vi "T_CAN CONF.vi"() -> ()   [LabVIEW 2018]
uses:
  Controls/CLUSTER.ctl
  Controls/FEV_DBC CLUSTER.ctl
  Controls/DBC CLUSTER.ctl
  <resource>/objmgr/xnet.rc
panel:
  out "Signals":refnum<k21>[](array[refnum])
  in  "DBC FUNCTIONS":T1[](array[typedef])
  out "Headline":string
  in  "ADD":bool
  in  "Save Button":bool
  in  "ALL DBC FUNCTIONS":T3[](array[typedef])
  in  "DBC File Selection":refnum<k21>="CAN DATA"
  in  "MODEL SELECTION":string(combo)
  # "FUNCTIONS"
  # "FUNCTIONS"
  # "READ"
  # "WRITE"
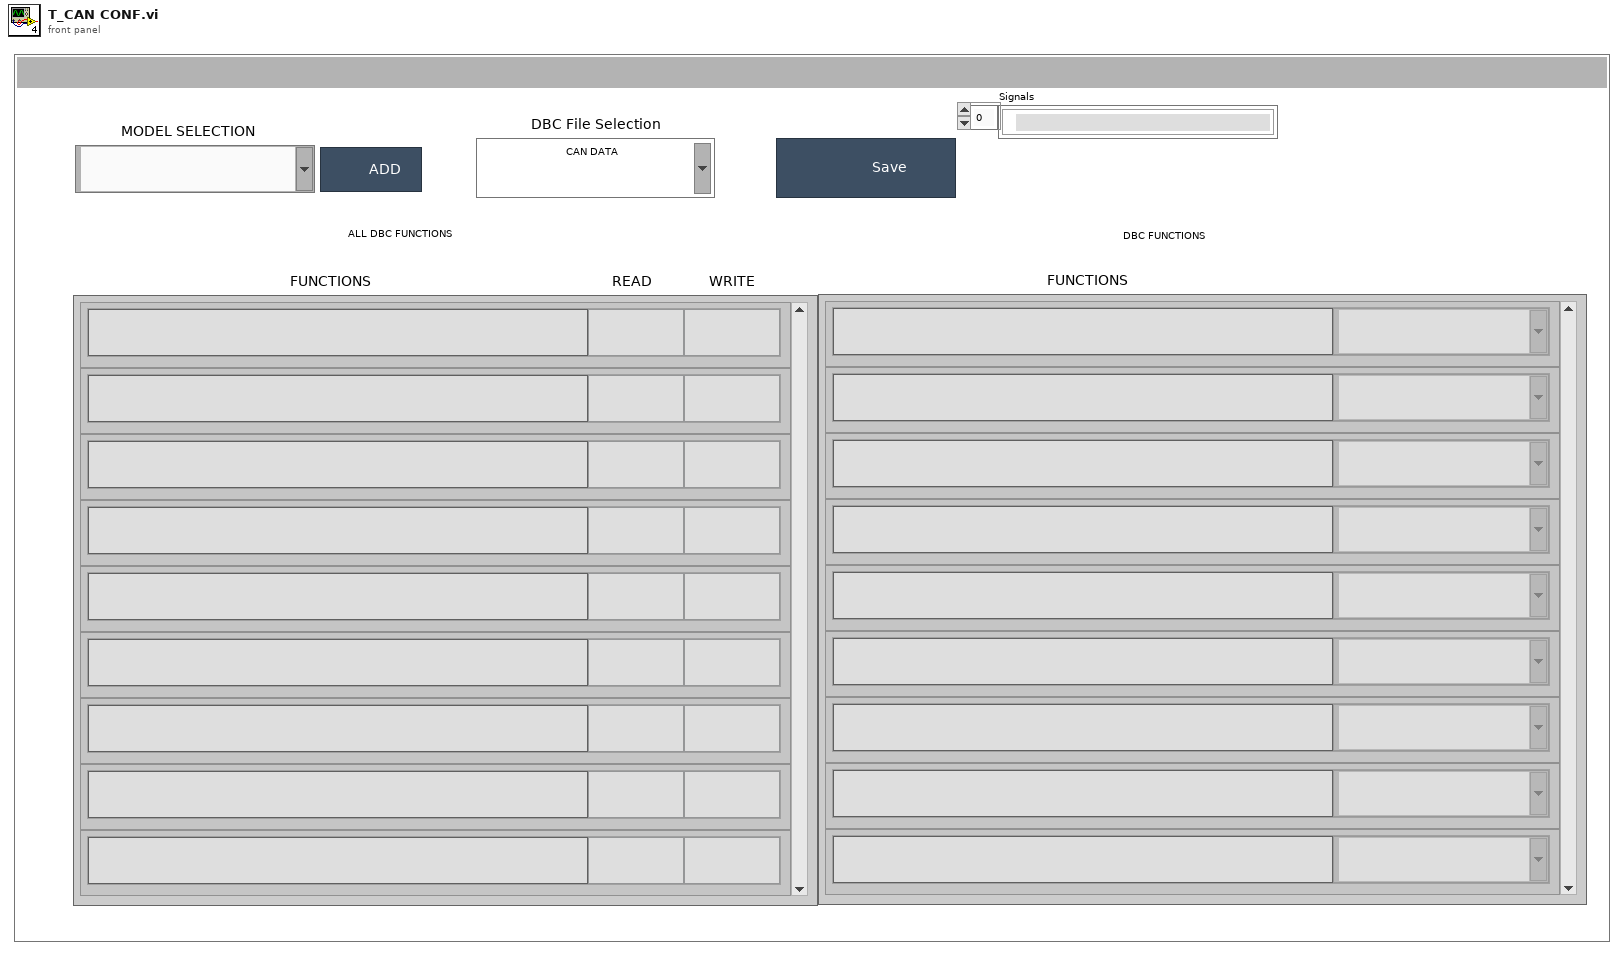
[diagram p1: front panel]
types:
  T1 = typedef "FEV_DBC CLUSTER.ctl" = cluster{"FUNCTION":T2, "DYNO FUNCTION":string}
  T2 = typedef "DBC CLUSTER.ctl" = string
  T3 = typedef "CLUSTER.ctl" = cluster{"FUNCTION":string, "READ":bool, "WRITE":bool}
  T4 = enum32{"Invalid", "Standard", "Closed", "Hidden", "Minimized", "Maximized"}
  T5 = enum32{"invalid app kind", "Development System", "Run Time System", "Student Edition", "Embedded LabVIEW", "Evaluation", "Custom"}
  T6 = cluster{"Core":cluster{"Current VI Reference":refnum<vi>, "Close Panel on Exit?":bool}, "Your Boolean data":bool, "Your string data":string, "ALL DBC FUNCTIONS":T3[], "File paths":cluster{"Base file path":path, "Model File path":path}, "DBC FUNCTIONS":T1[]}
  T7 = cluster{"Base file path":path, "Model File path":path}
  T8 = cluster{"Current VI Reference":refnum<vi>, "Close Panel on Exit?":bool}
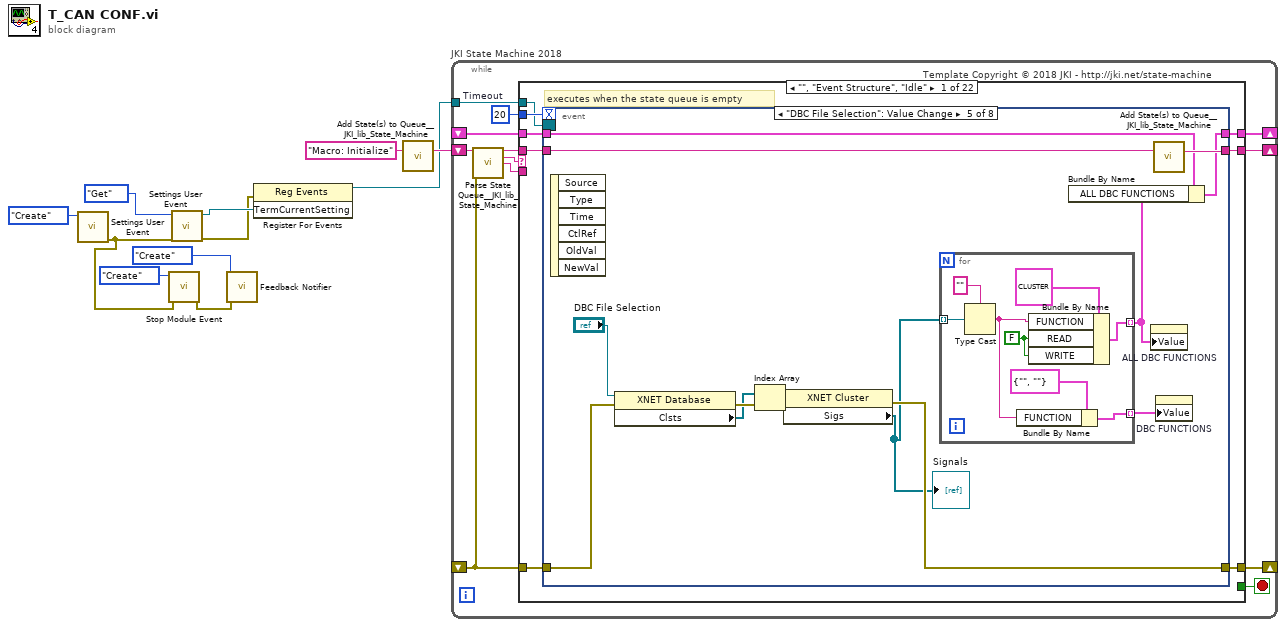
[diagram p0: block diagram]
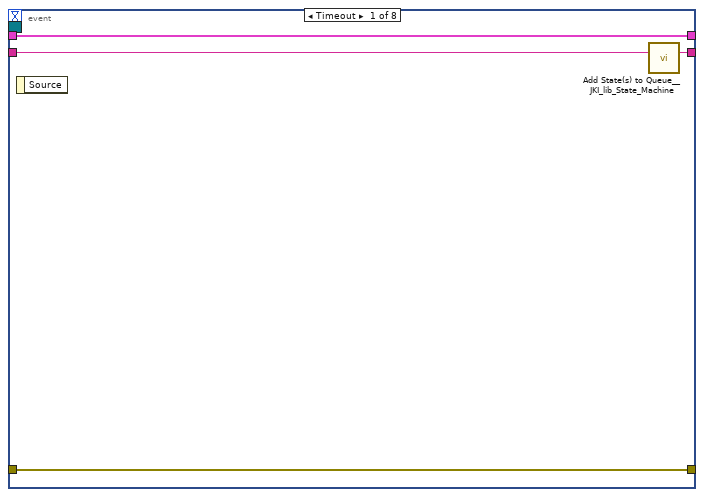
[diagram p2: hidden frame]
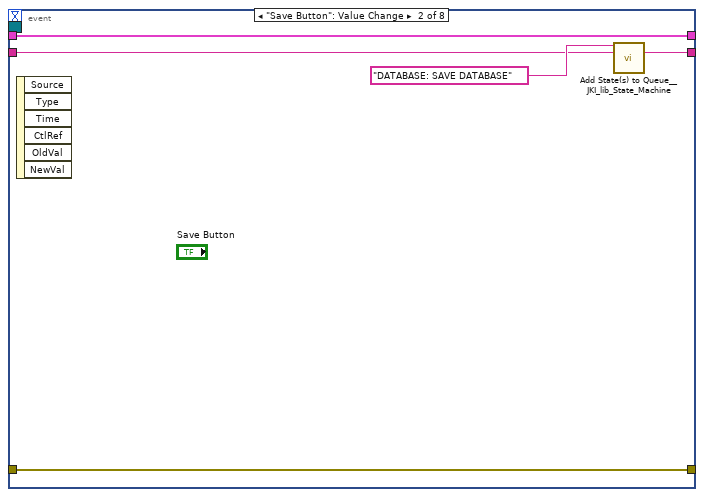
[diagram p3: hidden frame]
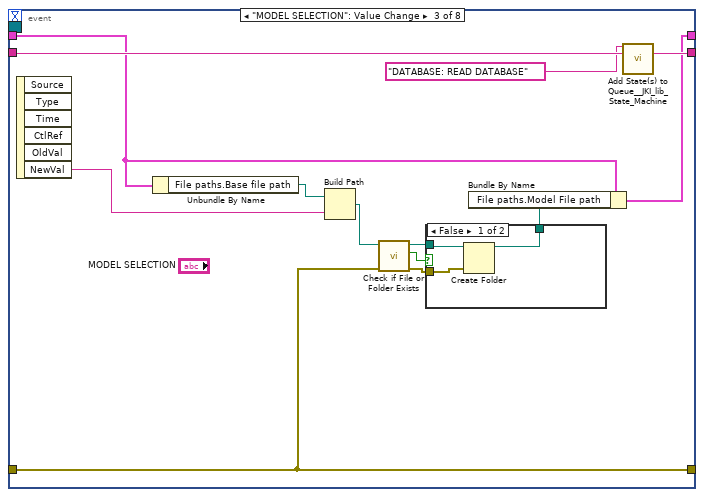
[diagram p4: hidden frame]
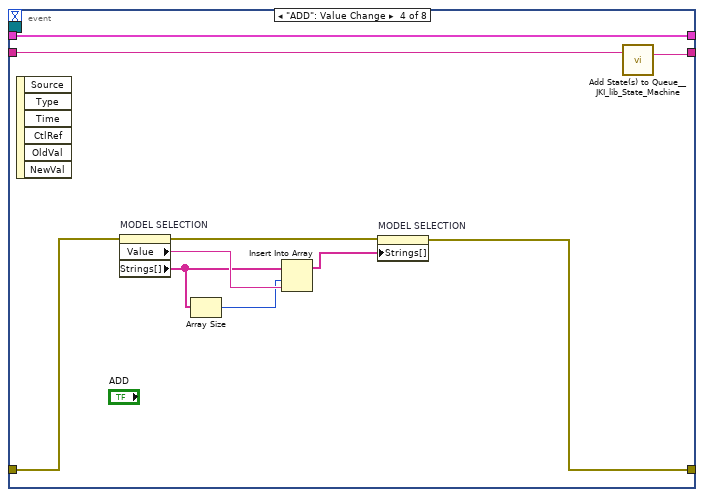
[diagram p6: hidden frame]
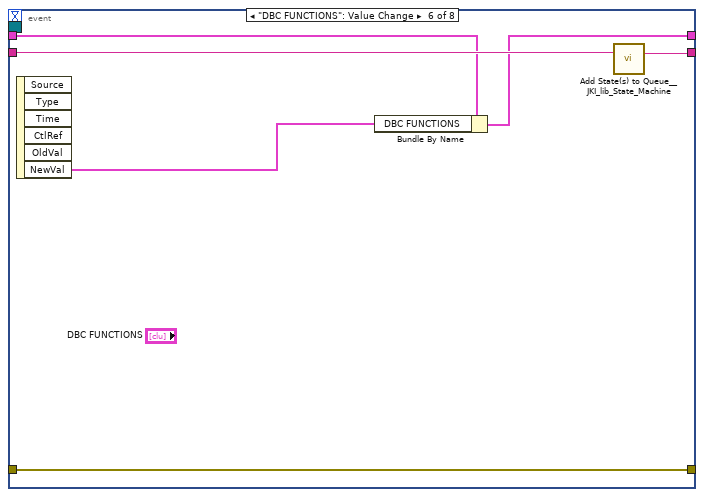
[diagram p7: hidden frame]
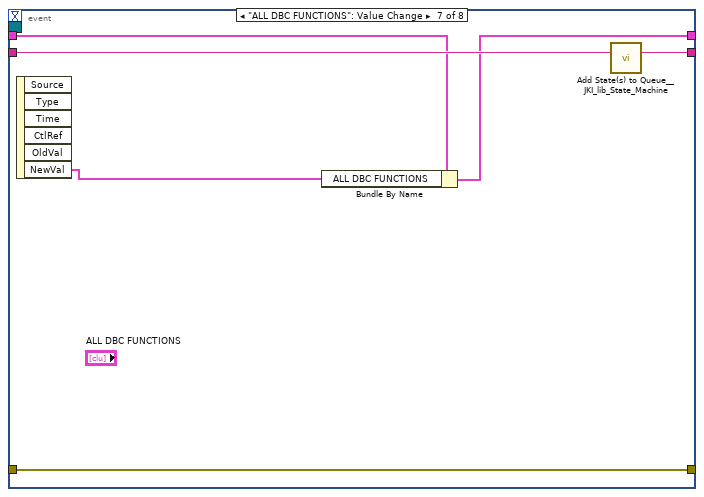
[diagram p8: hidden frame]
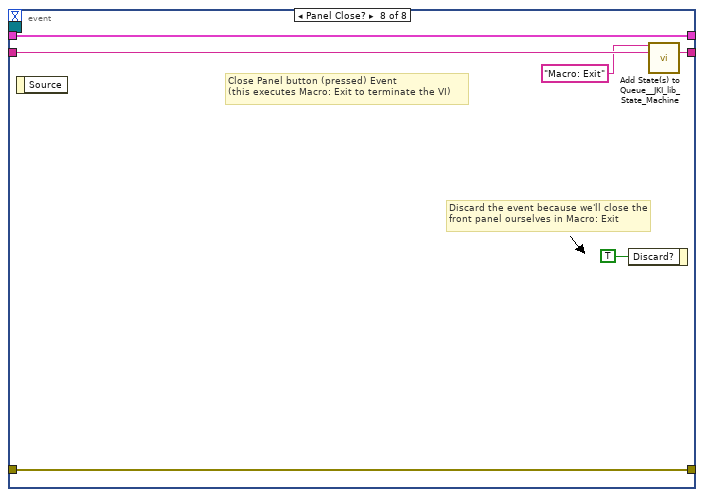
[diagram p9: hidden frame]
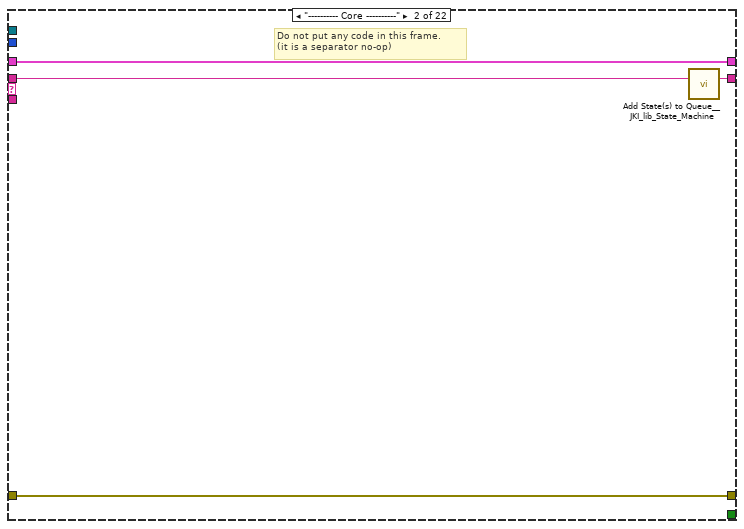
[diagram p10: hidden frame]
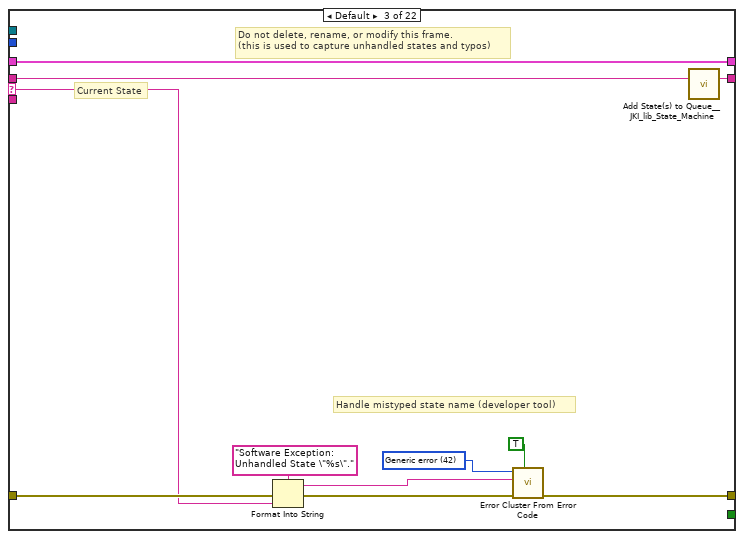
[diagram p11: hidden frame]
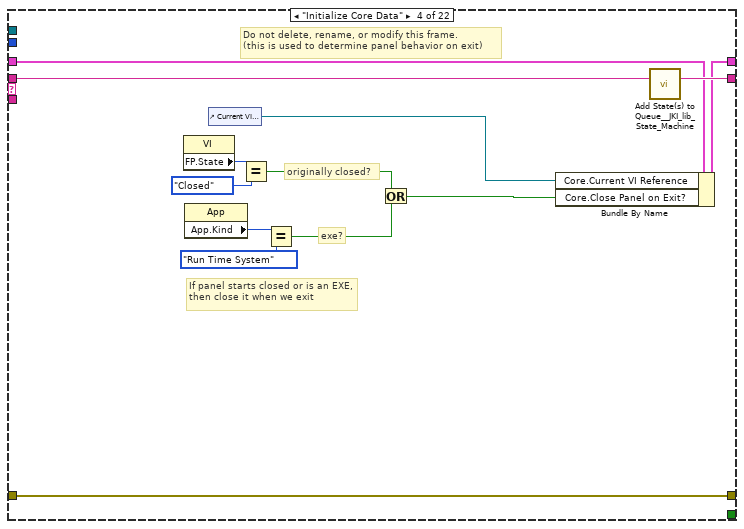
[diagram p12: hidden frame]
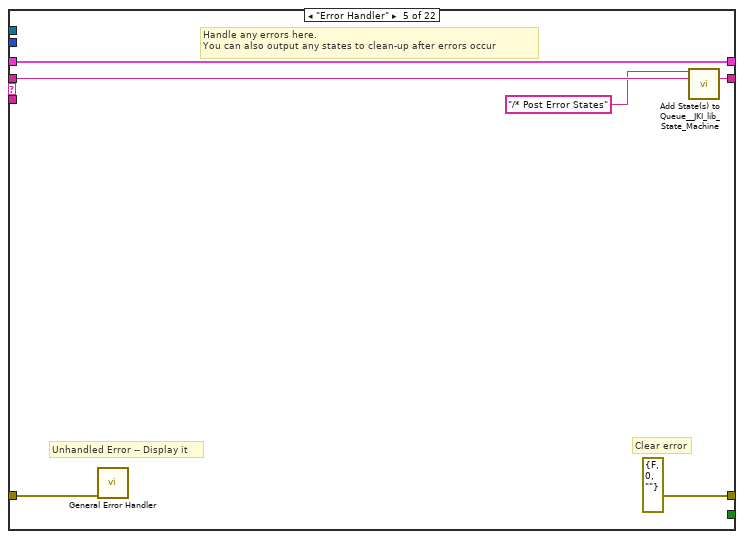
[diagram p13: hidden frame]
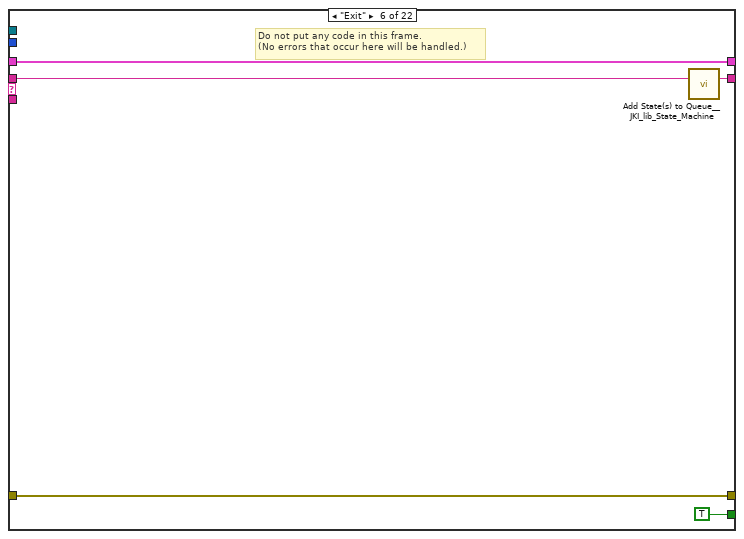
[diagram p14: hidden frame]
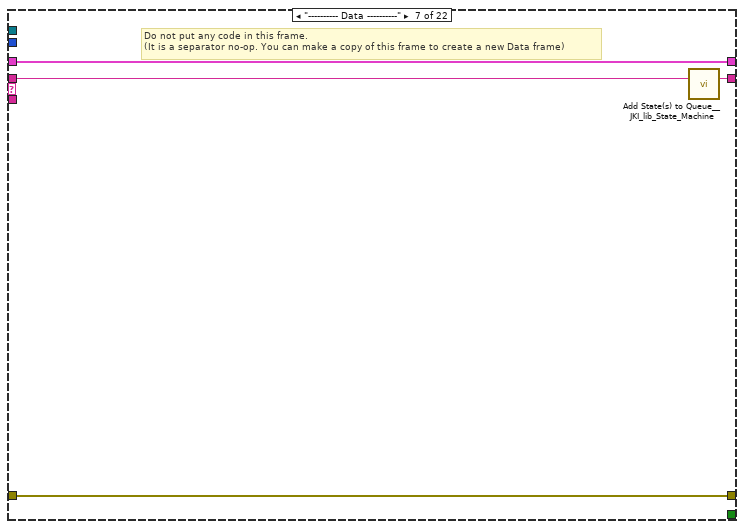
[diagram p15: hidden frame]
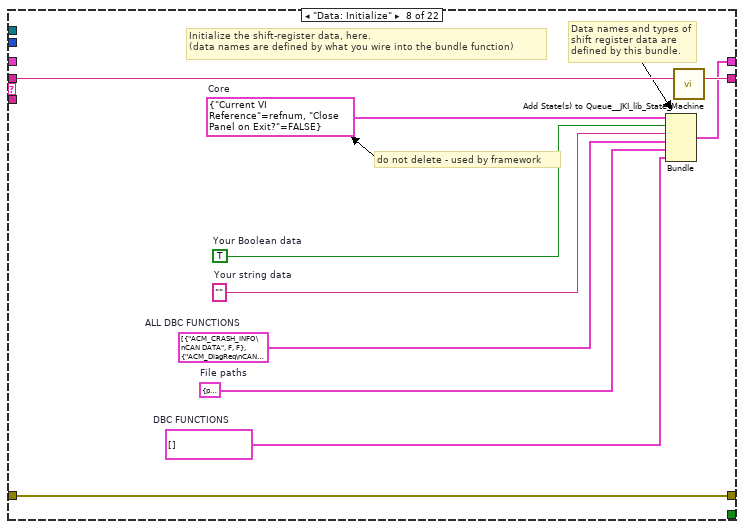
[diagram p16: hidden frame]
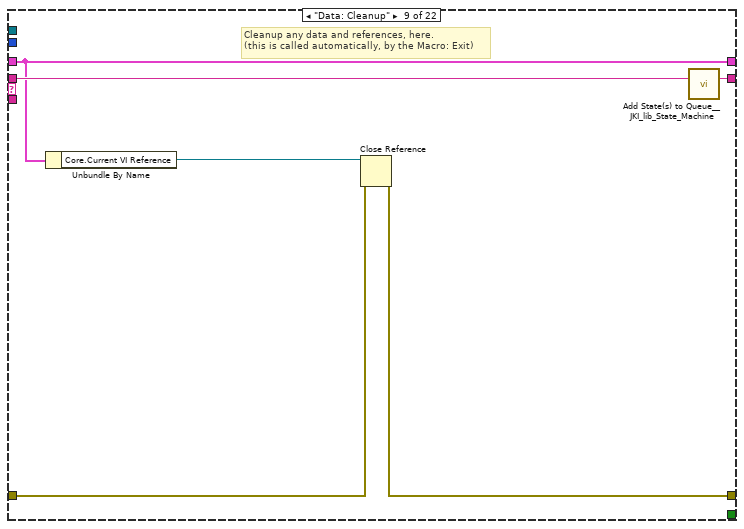
[diagram p17: hidden frame]
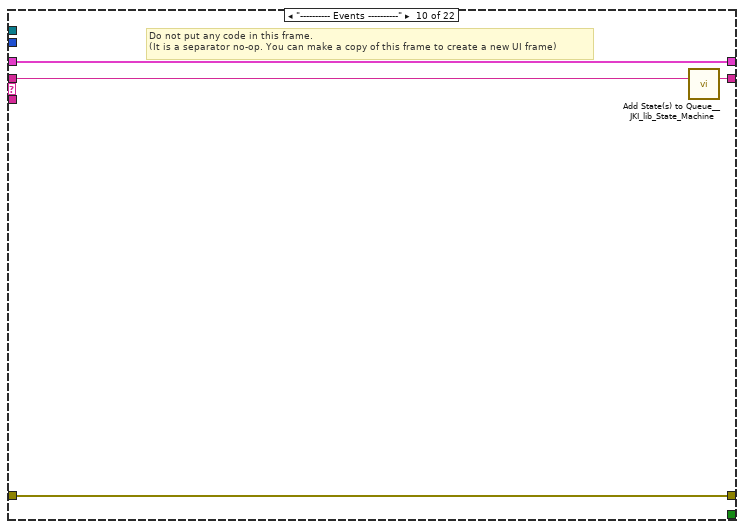
[diagram p18: hidden frame]
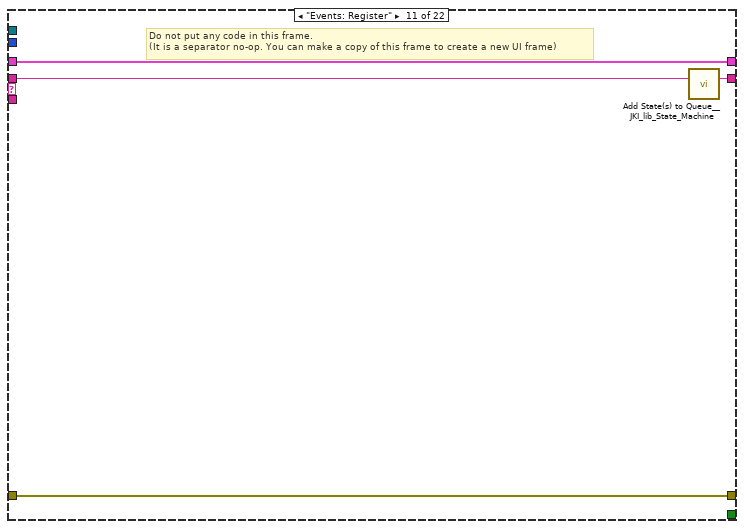
[diagram p19: hidden frame]
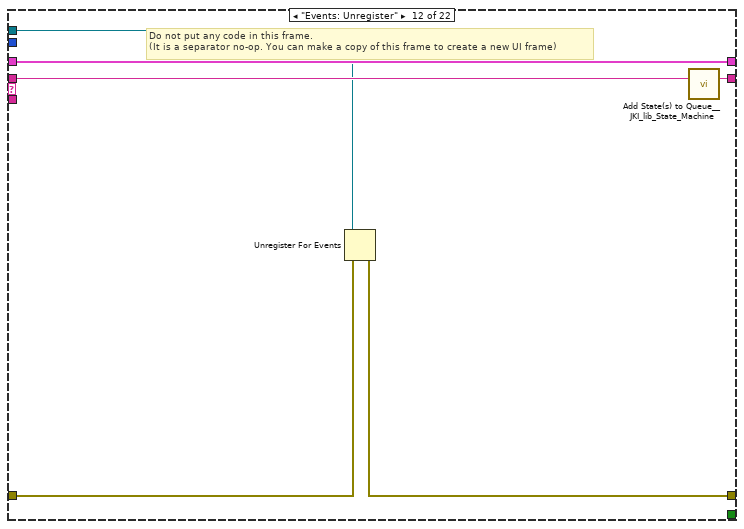
[diagram p20: hidden frame]
diagram:
  n1 = call "Settings User Event.vi"("Action"=enum16{"Create", "Get", "Destroy"}."Create") -> ("error out"=w4:errorcluster)  [unwired: 9 in, 1 out]
  n2 = call "Stop Module Event.vi"("error in (no error)"=w4, "Action"=enum16{"Create", "Get", "Destroy"}."Create") -> ("error out"=w3:errorcluster)  [unwired: 8 in, 1 out]
  n3 = call "Settings User Event.vi"("error in (no error)"=w4, "Action"=enum16{"Create", "Get", "Destroy"}."Get") -> ("error out"=w6:errorcluster, "TermCurrentSetting"=w7:refnum<user-event>)  [unwired: 8 in]
  n4 = call "Feedback Notifier.vi"("error in (no error)"=w3, "Action"=enum16{"Create", "Get", "Destroy"}."Create") -> ()  [unwired: 8 in, 2 out]
  n5 = register-events(error in=w6, w7) -> (reference out=w1:refnum<event-registration>)  [unwired: 1 in, 1 out]
  n6 = call <vilib>:"Add State(s) to Queue__JKI_lib_State_Machine.vi"("State(s) in (\"\")"="Macro: Initialize") -> ("States Out"=w11:string)  [unwired: 14 in]
  n7 = while "JKI State Machine 2018" {
    shift-right: [w16] -> _
    shift-left: _ -> [w15]
    shift-right: [w19] -> _
    shift-left: _ -> [w13]
    shift-right: [w18] -> _
    shift-left: w11 -> [w20]
    tunnel: w1 -> [w12]
    stop <- w17 stop-if-true
    w14 = 20  # Timeout
    # "Template Copyright © 2018 JKI - http://jki.net/state-machine"
    n8 = call <vilib>:"Parse State Queue__JKI_lib_State_Machine.vi"("State Queue"=w20, "Error In (no error)"=w13) -> ("Remaining States"=w22:string, "Current State"=w23:string, "Arguments"=w21:string)  [unwired: 11 in]
    n9 = case shown="\"\", \"Event Structure\", \"Idle\"" w23 {
      selector: w23 -> [_ _ w111 _ _ _ _ _ _ _ _ _ _ _ _ _ _ _ _ _ _ _]
      tunnel: w22 -> [w31 w110 w115 w134 w140 w145 w149 w159 w165 w169 w173 w179 w183 w195 w201 w212 w281 w286 w296 w300 w314 w337]
      tunnel: w21 -> [_ _ _ _ _ _ _ _ _ _ _ _ _ _ w196 w206 _ _ _ _ _ _]
      tunnel: w15 -> [w29 w107 w113 w127 w137 w143 w146 _ w160 w166 w171 w177 w180 w189 w199 w208 w278 w283 w293 w297 w312 w333]
      tunnel: [w28 w108 w117 w131 errorcluster {"status"=FALSE, "code"=0, "source"=""} ("error out") w142 w147 w156 w161 w167 w170 w174 w181 w190 w197 w209 w279 w284 w294 w298 w302 w331] -> w19
      tunnel: w13 -> [w27 w108 w116 w131 w136 w142 w147 w156 w162 w167 w170 w175 w181 w186 w198 w210 w279 w284 w294 w298 w311 w322]
      tunnel: [w30 w109 w114 w133 w139 w144 w148 w158 w164 w168 w172 w178 w182 w194 w200 w211 w280 w285 w295 w299 w313 w336] -> w18
      tunnel: [_ _ _ _ _ TRUE _ _ _ _ _ _ _ _ _ _ _ _ _ _ _ _] -> w17
      tunnel: [w26 w107 w113 w132 w137 w143 w146 w157 w160 w166 w171 w177 w180 w188 w199 w208 w278 w283 w293 w297 w312 w332] -> w16
      tunnel: w14 -> [w25 _ _ _ _ _ _ _ _ _ _ _ _ _ _ _ _ _ _ _ _ _]
      tunnel: w12 -> [w24 _ _ _ _ _ _ _ _ _ _ w176 _ _ _ _ _ _ _ _ _ _]
      frame "", "Event Structure", "Idle" {
        # "executes when the state queue is empty"
        n10 = event shown="[4] \"DBC File Selection\": Value Change" {
          selector: w24 -> [_ _ _ _ _ _ _ _]
          dyn-events: _ -> [_ _ _ _ _ _ _ _]
          timeout: w25 -> [_ _ _ _ _ _ _ _]
          tunnel: w31 -> [w35 w37 w52 w58 w73 w92 w98 w106]
          tunnel: [w34 w38 w53 w59 w74 w93 w99 w105] -> w30
          tunnel: w29 -> [w32 w39 w48 w60 w72 w91 w97 w103]
          tunnel: [w33 w36 w45 w61 w75 w94 w100 w104] -> w28
          tunnel: w27 -> [w33 w36 w45 w67 w76 w94 w100 w104]
          tunnel: [w32 w39 w47 w60 w71 w89 w95 w103] -> w26
          event Timeout {
            n11 = event-data() -> ()  [unwired: 1 in, 1 out]
            n12 = call <vilib>:"Add State(s) to Queue__JKI_lib_State_Machine.vi"("State(s) in (\"\")"=w35) -> ("States Out"=w34:string)  [unwired: 14 in]
          }
          event "Save Button": Value Change {
            n13 = event-data() -> ()  [unwired: 1 in, 6 out]
            n14 = call <vilib>:"Add State(s) to Queue__JKI_lib_State_Machine.vi"("State(s) in Front (\"\")"="DATABASE: SAVE DATABASE", "State(s) in (\"\")"=w37) -> ("States Out"=w38:string)  [unwired: 13 in]
          }
          event "MODEL SELECTION": Value Change {
            n15 = event-data() -> ("NewVal"=w49:string)  [unwired: 1 in, 5 out]
            n16 = Unbundle By Name(w48) -> ("File paths.Base file path"=w50:path)
            n17 = Build Path(base path=w50, name or relative path=w49) -> (appended path=w46:path)
            n18 = call <vilib>:"Check if File or Folder Exists.vi"("error in (no error)"=w45, "path"=w46) -> ("error out"=w43:errorcluster, "file or folder exists?"=w42:bool, "dup path"=w44:path)  [unwired: 7 in]
            n19 = case shown="False" w42 {
              tunnel: w44 -> [w55 w57]
              tunnel: w43 -> [w56 _]
              tunnel: [w54 w57] -> w41
              frame False {
                n20 = Create Folder(path (use dialog)=w55, error in=w56) -> (created path=w54:path)  [unwired: 1 in, 2 out]
              }
              frame True {
              }
            }
            n21 = Bundle By Name(cluster=w48, "File paths.Model File path"=w41) -> (w47:T6)
            n22 = call <vilib>:"Add State(s) to Queue__JKI_lib_State_Machine.vi"("State(s) in Front (\"\")"="DATABASE: READ DATABASE", "State(s) in (\"\")"=w52) -> ("States Out"=w53:string)  [unwired: 13 in]
          }
          event "ADD": Value Change {
            n23 = event-data() -> ()  [unwired: 1 in, 6 out]
            n24 = property on="MODEL SELECTION" class="CmbBox"(error in=w67) -> (error out=w66:errorcluster, "Value"=w65:string, "Strings[]"=w64:string[])  [unwired: 1 in, 1 out]
            n25 = Array Size(array=w64) -> (size(s)=w63:i32)
            n26 = Insert Into Array(array=w64, index=w63, new element=w65) -> (w62:string[])
            n27 = property on="MODEL SELECTION" class="CmbBox"(error in=w66, "Strings[]"=w62) -> (error out=w61:errorcluster)  [unwired: 1 in, 1 out]
            n28 = call <vilib>:"Add State(s) to Queue__JKI_lib_State_Machine.vi"("State(s) in (\"\")"=w58) -> ("States Out"=w59:string)  [unwired: 14 in]
          }
          event "DBC File Selection": Value Change {
            n29 = event-data() -> ()  [unwired: 1 in, 6 out]
            n30 = property class="XNET Database"(reference="DBC File Selection", error in=w76) -> (error out=w79:errorcluster, "Clsts"=w78:refnum<k21>[])  [unwired: 1 out]
            n31 = Index Array(array=w78) -> (element=w80:refnum<k21>)  [unwired: 1 in]
            n32 = property class="XNET Cluster"(reference=w80, error in=w79) -> (error out=w75:errorcluster, "Sigs"=w68:refnum<k21>[])  [unwired: 1 out]
            "Signals" <- w68
            n33 = for {
              tunnel: [w87] -> w70 mode=indexing
              tunnel: w68 -> [w84] mode=indexing
              tunnel: [w81] -> w69 mode=indexing
              w85 = FALSE ("READ")
              n34 = Type Cast(type="" ("FUNCTION"), x=w84) -> (*(type *) &x=w82:string)
              n35 = Bundle By Name(cluster=T1 {"FUNCTION"="", "DYNO FUNCTION"=""} ("FUNCTIONS"), "FUNCTION"=w82) -> (w81:T1)
              n36 = Bundle By Name(cluster=T3 {"FUNCTION"="ACM_CRASH_INFO\nCAN DATA", "READ"=TRUE, "WRITE"=TRUE} ("FUNCTIONS"), "FUNCTION"=w82, "READ"=w85, "WRITE"=w85) -> (w87:T3)
            }
            n37 = Bundle By Name(cluster=w72, "ALL DBC FUNCTIONS"=w70) -> (w71:T6)
            n38 = property on="ALL DBC FUNCTIONS" class="Arr (strict)"("Value"=w70) -> ()  [unwired: 2 in, 2 out]
            n39 = call <vilib>:"Add State(s) to Queue__JKI_lib_State_Machine.vi"("State(s) in (\"\")"=w73) -> ("States Out"=w74:string)  [unwired: 14 in]
            n40 = property on="DBC FUNCTIONS" class="Arr (strict)"("Value"=w69) -> ()  [unwired: 2 in, 2 out]
          }
          event "DBC FUNCTIONS": Value Change {
            n41 = event-data() -> ("NewVal"=w90:T1[])  [unwired: 1 in, 5 out]
            n42 = Bundle By Name(cluster=w91, "DBC FUNCTIONS"=w90) -> (w89:T6)
            n43 = call <vilib>:"Add State(s) to Queue__JKI_lib_State_Machine.vi"("State(s) in (\"\")"=w92) -> ("States Out"=w93:string)  [unwired: 14 in]
          }
          event "ALL DBC FUNCTIONS": Value Change {
            n44 = event-data() -> ("NewVal"=w96:T3[])  [unwired: 1 in, 5 out]
            n45 = Bundle By Name(cluster=w97, "ALL DBC FUNCTIONS"=w96) -> (w95:T6)
            n46 = call <vilib>:"Add State(s) to Queue__JKI_lib_State_Machine.vi"("State(s) in (\"\")"=w98) -> ("States Out"=w99:string)  [unwired: 14 in]
          }
          event Panel Close? {
            # "Discard the event because we'll close the front panel ourselves in Macro: Exit"
            # "Close Panel button (pressed) Event\n(this executes Macro: Exit to terminate the VI)"
            n47 = event-data() -> ()  [unwired: 1 in, 1 out]
            n48 = event-data("Discard?"=TRUE) -> ()  [unwired: 1 in, 1 out]
            n49 = call <vilib>:"Add State(s) to Queue__JKI_lib_State_Machine.vi"("State(s) in Front (\"\")"="Macro: Exit", "State(s) in (\"\")"=w106) -> ("States Out"=w105:string)  [unwired: 13 in]
          }
        }
      }
      frame "---------- Core ----------" {
        # "Do not put any code in this frame.\n(it is a separator no-op)"
        n50 = call <vilib>:"Add State(s) to Queue__JKI_lib_State_Machine.vi"("State(s) in (\"\")"=w110) -> ("States Out"=w109:string)  [unwired: 14 in]
      }
      frame Default {
        w120 = 42 items=["No error", "Argument error", "Memory is full", "Out of zone", "End of file", "File already open", "Generic file I/O error", "File not found", "File permission error", "Disk is full", "Duplicate path", "Too many files open", "System feature not enabled", "Resource file not found", "Cannot add resource", "Resource not found", "Image not found", "Image memory error", "Pen does not exist", "Config type invalid", "Config token not found", "Config parse error", "Config memory error", "Bad external code format", "Bad external code offset", "External code not present", "Null window", "Destroy window error", "Null menu", "Print aborted", "Bad print record", "Print driver error", "Windows error during printing", "Memory error during printing", "Print dialog error", "Generic print error", "Invalid device refnum", "Device not found", "Device parameter error", "Device unit error", "Cannot open device", "Device call aborted", "Generic error", "Cancelled by user", "Object ID too low", "Object ID too high", "Object not in heap", "Unknown heap", "Unknown object (invalid DefProc)", "Unknown object (DefProc not in table)", "Message out of range", "Invalid (null) method", "Unknown message", "Manager call not supported", "Bad address", "Network operation in progress", "Network operation timed out", "Connection is busy", "Network attribute not supported", "Network error", "Address in use", "System out of memory", "Connection aborted", "Connection refused", "Not connected", "Already connected", "Connection closed", "Initialization error (interapplication manager)", "Bad occurrence", "Wait on unbound occurrence handler", "Occurrence queue overflow", "Datalog type conflict", "Unused", "Unrecognized type (interapplication manager)", "Memory corrupt", "Failed to make temporary DLL", "Old CIN version", "Drag socket not found", "Failed to load drop-object", "Failed to register OLE object", "Failed to release OLE object", "Format specifier type mismatch", "Unknown format specifier", "Too few format specifiers", "Too many format specifiers", "Scan failed", "Newer CIN version", "Error converting to variant", "Runtime menu error", "Password tampered", "Variant attribute not found", "Incompatible variant data type", "Event data is not available", "Event Store is not present", "Occurrence is not found", "Event Queue is not created", "Event info is not available", "Refnum passed is NULL", "Error retrieving Class GUID", "Error retrieving CoClass GUID", "Error retrieving TypeLib GUID.", "Bad built application magic bytes.", "Specific driver is different from the specific driver associated with the Logical Name.", "There is no session opened to the class driver.", "Max Error", "MAX - Error with config objects", "MAX - Error loading configuration", "MAX - Group not supported"]
        # "Current State"
        # "Do not delete, rename, or modify this frame.\n(this is used to capture unhandled states and typos)"
        # "Handle mistyped state name (developer tool)"
        n51 = Format Into String(format string="Software Exception: Unhandled State \"%s\"." ("message"), error in=w116, w111) -> (resulting string=w119:string, error out=w118:errorcluster)  [unwired: 1 in]
        n52 = call <vilib>:"Error Cluster From Error Code.vi"("show call chain? (False)"=TRUE, "error in (no error)"=w118, "error message (\"\")"=w119, "error code (0)"=w120) -> ("error out"=w117:errorcluster)  [unwired: 5 in]
        n53 = call <vilib>:"Add State(s) to Queue__JKI_lib_State_Machine.vi"("State(s) in (\"\")"=w115) -> ("States Out"=w114:string)  [unwired: 14 in]
      }
      frame "Initialize Core Data" {
        # "Do not delete, rename, or modify this frame.\n(this is used to determine panel behavior on exit)"
        # "originally closed?"
        # "exe?"
        # "If panel starts closed or is an EXE, then close it when we exit"
        n54 = property class="VI"() -> ("FP.State"=w124:T4)  [unwired: 2 in, 2 out]
        n55 = property class="App"() -> ("App.Kind"=w130:T5)  [unwired: 2 in, 2 out]
        n56 = control-ref of="Current VI Reference"() -> (w125:refnum<vi>)
        n57 = Equal?(x=w124, y=T4."Closed" ("Front Panel Window:State")) -> (x = y?=w122:bool)
        n58 = Equal?(x=w130, y=T5."Run Time System" ("Application:Kind")) -> (x = y?=w128:bool)
        n59 = Or(x=w122, y=w128) -> (x .or. y?=w126:bool)
        n60 = Bundle By Name(cluster=w127, "Core.Current VI Reference"=w125, "Core.Close Panel on Exit?"=w126) -> (w132:T6)
        n61 = call <vilib>:"Add State(s) to Queue__JKI_lib_State_Machine.vi"("State(s) in (\"\")"=w134) -> ("States Out"=w133:string)  [unwired: 14 in]
      }
      frame "Error Handler" {
        # "Unhandled Error -- Display it"
        # "Handle any errors here.\nYou can also output any states to clean-up after errors occur"
        # "Clear error"
        n62 = call <vilib>:"General Error Handler.vi"("error in (no error)"=w136) -> ()  [unwired: 10 in, 5 out]
        n63 = call <vilib>:"Add State(s) to Queue__JKI_lib_State_Machine.vi"("State(s) in Front (\"\")"="/* Post Error States", "State(s) in (\"\")"=w140) -> ("States Out"=w139:string)  [unwired: 13 in]
      }
      frame "Exit" {
        # "Do not put any code in this frame.\n(No errors that occur here will be handled.)"
        n64 = call <vilib>:"Add State(s) to Queue__JKI_lib_State_Machine.vi"("State(s) in (\"\")"=w145) -> ("States Out"=w144:string)  [unwired: 14 in]
      }
      frame "---------- Data ----------" {
        # "Do not put any code in this frame.\n(It is a separator no-op. You can make a copy of this frame to create a new Data frame)"
        n65 = call <vilib>:"Add State(s) to Queue__JKI_lib_State_Machine.vi"("State(s) in (\"\")"=w149) -> ("States Out"=w148:string)  [unwired: 14 in]
      }
      frame "Data: Initialize" {
        w150 = T1[] []  # DBC FUNCTIONS
        w151 = T7 {"Base file path"=path "", "Model File path"=path ""}  # File paths
        w152 = T3[] [{"FUNCTION"="ACM_CRASH_INFO\nCAN DATA", "READ"=FALSE, "WRITE"=FALSE}, {"FUNCTION"="ACM_DiagReq\nCAN DATA", "READ"=FALSE, "WRITE"=FALSE}, {"FUNCTION"="ACM_DiagResp\nCAN DATA", "READ"=FALSE, "WRITE"=FALSE}, {"FUNCTION"="ACM_OCCUPANT_STATUS\nCAN DATA", "READ"=FALSE, "WRITE"=FALSE}, {"FUNCTION"="ACM_WarnMsg\nCAN DATA", "READ"=FALSE, "WRITE"=FALSE}, {"FUNCTION"="ADAS_AEB\nCAN DATA", "READ"=FALSE, "WRITE"=FALSE}, {"FUNCTION"="ADAS_AHB_DOW\nCAN DATA", "READ"=FALSE, "WRITE"=FALSE}, {"FUNCTION"="ADAS_APA_SLOT1INFO1\nCAN DATA", "READ"=FALSE, "WRITE"=FALSE}, {"FUNCTION"="ADAS_APA_SLOT1INFO2\nCAN DATA", "READ"=FALSE, "WRITE"=FALSE}, {"FUNCTION"="ADAS_APA_SLOT1INFO3\nCAN DATA", "READ"=FALSE, "WRITE"=FALSE}, {"FUNCTION"="ADAS_APA_SLOT2INFO1\nCAN DATA", "READ"=FALSE, "WRITE"=FALSE}, {"FUNCTION"="ADAS_APA_SLOT2INFO2\nCAN DATA", "READ"=FALSE, "WRITE"=FALSE}, {"FUNCTION"="ADAS_APA_SLOT2INFO3\nCAN DATA", "READ"=FALSE, "WRITE"=FALSE}, {"FUNCTION"="ADAS_APA_SLOT3INFO1\nCAN DATA", "READ"=FALSE, "WRITE"=FALSE}, {"FUNCTION"="ADAS_APA_SLOT3INFO2\nCAN DATA", "READ"=FALSE, "WRITE"=FALSE}, {"FUNCTION"="ADAS_APA_SLOT3INFO3\nCAN DATA", "READ"=FALSE, "WRITE"=FALSE}, {"FUNCTION"="ADAS_APA_SLOT4INFO1\nCAN DATA", "READ"=FALSE, "WRITE"=FALSE}, {"FUNCTION"="ADAS_APA_SLOT4INFO2\nCAN DATA", "READ"=FALSE, "WRITE"=FALSE}, {"FUNCTION"="ADAS_APA_SLOT4INFO3\nCAN DATA", "READ"=FALSE, "WRITE"=FALSE}, {"FUNCTION"="ADAS_APA_SLOT5INFO1\nCAN DATA", "READ"=FALSE, "WRITE"=FALSE}, {"FUNCTION"="ADAS_APA_SLOT5INFO2\nCAN DATA", "READ"=FALSE, "WRITE"=FALSE}, {"FUNCTION"="ADAS_APA_SLOT5INFO3\nCAN DATA", "READ"=FALSE, "WRITE"=FALSE}, {"FUNCTION"="ADAS_APA_SLOT6INFO1\nCAN DATA", "READ"=FALSE, "WRITE"=FALSE}, {"FUNCTION"="ADAS_APA_SLOT6INFO2\nCAN DATA", "READ"=FALSE, "WRITE"=FALSE}, {"FUNCTION"="ADAS_APA_SLOT6INFO3\nCAN DATA", "READ"=FALSE, "WRITE"=FALSE}, {"FUNCTION"="ADAS_AVM_Sts\nCAN DATA", "READ"=FALSE, "WRITE"=FALSE}, {"FUNCTION"="ADAS_BSD\nCAN DATA", "READ"=FALSE, "WRITE"=FALSE}, {"FUNCTION"="ADAS_CMP_ACC\nCAN DATA", "READ"=FALSE, "WRITE"=FALSE}, {"FUNCTION"="ADAS_CMP_CHECK\nCAN DATA", "READ"=FALSE, "WRITE"=FALSE}, {"FUNCTION"="ADAS_CMP_MHU\nCAN DATA", "READ"=FALSE, "WRITE"=FALSE}, {"FUNCTION"="ADAS_DMS_STATUS\nCAN DATA", "READ"=FALSE, "WRITE"=FALSE}, {"FUNCTION"="ADAS_DiagReq\nCAN DATA", "READ"=FALSE, "WRITE"=FALSE}, {"FUNCTION"="ADAS_DiagResp\nCAN DATA", "READ"=FALSE, "WRITE"=FALSE}, {"FUNCTION"="ADAS_ELK\nCAN DATA", "READ"=FALSE, "WRITE"=FALSE}, {"FUNCTION"="ADAS_FCW_RCTA\nCAN DATA", "READ"=FALSE, "WRITE"=FALSE}, {"FUNCTION"="ADAS_Immo_MHU\nCAN DATA", "READ"=FALSE, "WRITE"=FALSE}, {"FUNCTION"="ADAS_LDW_LKA\nCAN DATA", "READ"=FALSE, "WRITE"=FALSE}, {"FUNCTION"="ADAS_NM\nCAN DATA", "READ"=FALSE, "WRITE"=FALSE}, {"FUNCTION"="ADAS_PA\nCAN DATA", "READ"=FALSE, "WRITE"=FALSE}, {"FUNCTION"="ADAS_RP_Sts\nCAN DATA", "READ"=FALSE, "WRITE"=FALSE}, {"FUNCTION"="ADAS_Speed_Display\nCAN DATA", "READ"=FALSE, "WRITE"=FALSE}, {"FUNCTION"="ADAS_TSR_STATUS\nCAN DATA", "READ"=FALSE, "WRITE"=FALSE}, {"FUNCTION"="ADAS_WarnMsg\nCAN DATA", "READ"=FALSE, "WRITE"=FALSE}, {"FUNCTION"="AMP_DiagReq\nCAN DATA", "READ"=FALSE, "WRITE"=FALSE}, {"FUNCTION"="AMP_DiagResp\nCAN DATA", "READ"=FALSE, "WRITE"=FALSE}, {"FUNCTION"="AMP_MHUEQType\nCAN DATA", "READ"=FALSE, "WRITE"=FALSE}, {"FUNCTION"="AMP_MHU_Ann1_ModeSET\nCAN DATA", "READ"=FALSE, "WRITE"=FALSE}, {"FUNCTION"="AMP_MHU_Ann1_PromptsSET\nCAN DATA", "READ"=FALSE, "WRITE"=FALSE}, {"FUNCTION"="AMP_MHU_Ann2_SpeakerSET\nCAN DATA", "READ"=FALSE, "WRITE"=FALSE}, {"FUNCTION"="AMP_MHU_SET\nCAN DATA", "READ"=FALSE, "WRITE"=FALSE}, {"FUNCTION"="AMP_NM\nCAN DATA", "READ"=FALSE, "WRITE"=FALSE}, {"FUNCTION"="AMP_rDiagReq\nCAN DATA", "READ"=FALSE, "WRITE"=FALSE}, {"FUNCTION"="AMP_rDiagResp\nCAN DATA", "READ"=FALSE, "WRITE"=FALSE}, {"FUNCTION"="APA_FEEDBACK_MHU\nCAN DATA", "READ"=FALSE, "WRITE"=FALSE}, {"FUNCTION"="APA_SENSOR\nCAN DATA", "READ"=FALSE, "WRITE"=FALSE}, {"FUNCTION"="APM_DiagReq\nCAN DATA", "READ"=FALSE, "WRITE"=FALSE}, {"FUNCTION"="APM_DiagResp\nCAN DATA", "READ"=FALSE, "WRITE"=FALSE}, {"FUNCTION"="APM_WINDOW_POS\nCAN DATA", "READ"=FALSE, "WRITE"=FALSE}, {"FUNCTION"="APM_WarnMsg\nCAN DATA", "READ"=FALSE, "WRITE"=FALSE}, {"FUNCTION"="ASU_DiagReq\nCAN DATA", "READ"=FALSE, "WRITE"=FALSE}, {"FUNCTION"="ASU_DiagResp\nCAN DATA", "READ"=FALSE, "WRITE"=FALSE}, {"FUNCTION"="AVAS_DiagReq\nCAN DATA", "READ"=FALSE, "WRITE"=FALSE}, {"FUNCTION"="AVAS_DiagResp\nCAN DATA", "READ"=FALSE, "WRITE"=FALSE}, {"FUNCTION"="AVAS_STATUS\nCAN DATA", "READ"=FALSE, "WRITE"=FALSE}, {"FUNCTION"="BCM_ALM_warning\nCAN DATA", "READ"=FALSE, "WRITE"=FALSE}, {"FUNCTION"="BCM_BPM_DiagReq\nCAN DATA", "READ"=FALSE, "WRITE"=FALSE}, {"FUNCTION"="BCM_BPM_DiagResp\nCAN DATA", "READ"=FALSE, "WRITE"=FALSE}, {"FUNCTION"="BCM_CLAMP_STAT\nCAN DATA", "READ"=FALSE, "WRITE"=FALSE}, {"FUNCTION"="BCM_Comfort_Confirm_sts\nCAN DATA", "READ"=FALSE, "WRITE"=FALSE}, {"FUNCTION"="BCM_DiagReq\nCAN DATA", "READ"=FALSE, "WRITE"=FALSE}, {"FUNCTION"="BCM_DiagResp\nCAN DATA", "READ"=FALSE, "WRITE"=FALSE}, {"FUNCTION"="BCM_ENERGY_MANAGEMENT\nCAN DATA", "READ"=FALSE, "WRITE"=FALSE}, {"FUNCTION"="BCM_ENTRY_CONTROL\nCAN DATA", "READ"=FALSE, "WRITE"=FALSE}, {"FUNCTION"="BCM_FKS_STATUS\nCAN DATA", "READ"=FALSE, "WRITE"=FALSE}, {"FUNCTION"="BCM_LIGHT\nCAN DATA", "READ"=FALSE, "WRITE"=FALSE}, {"FUNCTION"="BCM_LOGICAL_CLAMP\nCAN DATA", "READ"=FALSE, "WRITE"=FALSE}, {"FUNCTION"="BCM_Mirror_Confirm_sts\nCAN DATA", "READ"=FALSE, "WRITE"=FALSE}, {"FUNCTION"="BCM_ODO\nCAN DATA", "READ"=FALSE, "WRITE"=FALSE}, {"FUNCTION"="BCM_RainLightSnr\nCAN DATA", "READ"=FALSE, "WRITE"=FALSE}, {"FUNCTION"="BCM_SCM_LIN_Info\nCAN DATA", "READ"=FALSE, "WRITE"=FALSE}, {"FUNCTION"="BCM_STAT_CENTRAL_LOCK\nCAN DATA", "READ"=FALSE, "WRITE"=FALSE}, {"FUNCTION"="BCM_STAT_DOOR_FLAP\nCAN DATA", "READ"=FALSE, "WRITE"=FALSE}, {"FUNCTION"="BCM_SunroofSts\nCAN DATA", "READ"=FALSE, "WRITE"=FALSE}, {"FUNCTION"="BCM_SunshadeSts\nCAN DATA", "READ"=FALSE, "WRITE"=FALSE}, {"FUNCTION"="BCM_SwitchSts\nCAN DATA", "READ"=FALSE, "WRITE"=FALSE}, {"FUNCTION"="BCM_TERMINAL\nCAN DATA", "READ"=FALSE, "WRITE"=FALSE}, {"FUNCTION"="BCM_VEHICLE_IDENT_NUMBER\nCAN DATA", "READ"=FALSE, "WRITE"=FALSE}, {"FUNCTION"="BCM_VOLTAGE\nCAN DATA", "READ"=FALSE, "WRITE"=FALSE}, {"FUNCTION"="BCM_WarnMsg\nCAN DATA", "READ"=FALSE, "WRITE"=FALSE}, {"FUNCTION"="BMS_CellTemp\nCAN DATA", "READ"=FALSE, "WRITE"=FALSE}, {"FUNCTION"="BMS_ChgParamReq\nCAN DATA", "READ"=FALSE, "WRITE"=FALSE}, {"FUNCTION"="BMS_CurMeas\nCAN DATA", "READ"=FALSE, "WRITE"=FALSE}, {"FUNCTION"="BMS_DiagReq\nCAN DATA", "READ"=FALSE, "WRITE"=FALSE}, {"FUNCTION"="BMS_DiagResp\nCAN DATA", "READ"=FALSE, "WRITE"=FALSE}, {"FUNCTION"="BMS_HVMeas1\nCAN DATA", "READ"=FALSE, "WRITE"=FALSE}, {"FUNCTION"="BMS_Sts\nCAN DATA", "READ"=FALSE, "WRITE"=FALSE}, {"FUNCTION"="BMS_WarnMsg\nCAN DATA", "READ"=FALSE, "WRITE"=FALSE}, {"FUNCTION"="CCUF_DiagReq\nCAN DATA", "READ"=FALSE, "WRITE"=FALSE}, {"FUNCTION"="CCUF_DiagResp\nCAN DATA", "READ"=FALSE, "WRITE"=FALSE}, {"FUNCTION"="CCUR_DiagReq\nCAN DATA", "READ"=FALSE, "WRITE"=FALSE}, {"FUNCTION"="CCUR_DiagResp\nCAN DATA", "READ"=FALSE, "WRITE"=FALSE}, {"FUNCTION"="CCU_STATUS\nCAN DATA", "READ"=FALSE, "WRITE"=FALSE}, {"FUNCTION"="CCU_TEMP_PRESSURE\nCAN DATA", "READ"=FALSE, "WRITE"=FALSE}, {"FUNCTION"="CCU_WarnMsg\nCAN DATA", "READ"=FALSE, "WRITE"=FALSE}, {"FUNCTION"="CPD_DiagReq\nCAN DATA", "READ"=FALSE, "WRITE"=FALSE}, {"FUNCTION"="CPD_DiagResp\nCAN DATA", "READ"=FALSE, "WRITE"=FALSE}, {"FUNCTION"="CPD_NM\nCAN DATA", "READ"=FALSE, "WRITE"=FALSE}, {"FUNCTION"="CPD_OUTPUT\nCAN DATA", "READ"=FALSE, "WRITE"=FALSE}, {"FUNCTION"="CPD_WarnMsg\nCAN DATA", "READ"=FALSE, "WRITE"=FALSE}, {"FUNCTION"="CPD_rDiagReq\nCAN DATA", "READ"=FALSE, "WRITE"=FALSE}, {"FUNCTION"="CPD_rDiagResp\nCAN DATA", "READ"=FALSE, "WRITE"=FALSE}, {"FUNCTION"="Camera_Lane\nCAN DATA", "READ"=FALSE, "WRITE"=FALSE}, {"FUNCTION"="Camera_Object01\nCAN DATA", "READ"=FALSE, "WRITE"=FALSE}, {"FUNCTION"="Camera_Object02\nCAN DATA", "READ"=FALSE, "WRITE"=FALSE}, {"FUNCTION"="Camera_Object03\nCAN DATA", "READ"=FALSE, "WRITE"=FALSE}, {"FUNCTION"="Camera_Object04\nCAN DATA", "READ"=FALSE, "WRITE"=FALSE}, {"FUNCTION"="Camera_Object05\nCAN DATA", "READ"=FALSE, "WRITE"=FALSE}, {"FUNCTION"="Camera_Object06\nCAN DATA", "READ"=FALSE, "WRITE"=FALSE}, {"FUNCTION"="Camera_leftlane\nCAN DATA", "READ"=FALSE, "WRITE"=FALSE}, {"FUNCTION"="Camera_rightlane\nCAN DATA", "READ"=FALSE, "WRITE"=FALSE}, {"FUNCTION"="DCM_APM_DiagReq\nCAN DATA", "READ"=FALSE, "WRITE"=FALSE}, {"FUNCTION"="DCM_APM_DiagResp\nCAN DATA", "READ"=FALSE, "WRITE"=FALSE}, {"FUNCTION"="DIAG_Req_All_CAN\nCAN DATA", "READ"=FALSE, "WRITE"=FALSE}, {"FUNCTION"="DIAG_Req_All_Ecu\nCAN DATA", "READ"=FALSE, "WRITE"=FALSE}, {"FUNCTION"="DIAG_Req_Info\nCAN DATA", "READ"=FALSE, "WRITE"=FALSE}, {"FUNCTION"="DMS_Status\nCAN DATA", "READ"=FALSE, "WRITE"=FALSE}, {"FUNCTION"="Diag_Request_ECU\nCAN DATA", "READ"=FALSE, "WRITE"=FALSE}, {"FUNCTION"="EASC_Confirm_sts\nCAN DATA", "READ"=FALSE, "WRITE"=FALSE}, {"FUNCTION"="EASC_DiagReq\nCAN DATA", "READ"=FALSE, "WRITE"=FALSE}, {"FUNCTION"="EASC_DiagResp\nCAN DATA", "READ"=FALSE, "WRITE"=FALSE}, {"FUNCTION"="EASC_NM\nCAN DATA", "READ"=FALSE, "WRITE"=FALSE}, {"FUNCTION"="EASC_WarnMsg\nCAN DATA", "READ"=FALSE, "WRITE"=FALSE}, {"FUNCTION"="EASC_rDiagReq\nCAN DATA", "READ"=FALSE, "WRITE"=FALSE}, {"FUNCTION"="EASC_rDiagResp\nCAN DATA", "READ"=FALSE, "WRITE"=FALSE}, {"FUNCTION"="EDS_F_DiagReq\nCAN DATA", "READ"=FALSE, "WRITE"=FALSE}, {"FUNCTION"="EDS_F_DiagResp\nCAN DATA", "READ"=FALSE, "WRITE"=FALSE}, {"FUNCTION"="EDS_F_WarnMsg\nCAN DATA", "READ"=FALSE, "WRITE"=FALSE}, {"FUNCTION"="EDS_OutPut_FR\nCAN DATA", "READ"=FALSE, "WRITE"=FALSE}, {"FUNCTION"="EDS_OutPut_RR\nCAN DATA", "READ"=FALSE, "WRITE"=FALSE}, {"FUNCTION"="EDS_R_DiagReq\nCAN DATA", "READ"=FALSE, "WRITE"=FALSE}, {"FUNCTION"="EDS_R_DiagResp\nCAN DATA", "READ"=FALSE, "WRITE"=FALSE}, {"FUNCTION"="EDS_R_WarnMsg\nCAN DATA", "READ"=FALSE, "WRITE"=FALSE}, {"FUNCTION"="EPS2_DiagReq\nCAN DATA", "READ"=FALSE, "WRITE"=FALSE}, {"FUNCTION"="EPS2_DiagResp\nCAN DATA", "READ"=FALSE, "WRITE"=FALSE}, {"FUNCTION"="EPS_DiagReq\nCAN DATA", "READ"=FALSE, "WRITE"=FALSE}, {"FUNCTION"="EPS_DiagResp\nCAN DATA", "READ"=FALSE, "WRITE"=FALSE}, {"FUNCTION"="EPS_WarnMsg\nCAN DATA", "READ"=FALSE, "WRITE"=FALSE}, {"FUNCTION"="ETG_DiagReq\nCAN DATA", "READ"=FALSE, "WRITE"=FALSE}, {"FUNCTION"="ETG_DiagResp\nCAN DATA", "READ"=FALSE, "WRITE"=FALSE}, {"FUNCTION"="ETG_STATUS\nCAN DATA", "READ"=FALSE, "WRITE"=FALSE}, {"FUNCTION"="ETG_WarnMsg\nCAN DATA", "READ"=FALSE, "WRITE"=FALSE}, {"FUNCTION"="GS_DiagReq\nCAN DATA", "READ"=FALSE, "WRITE"=FALSE}, {"FUNCTION"="GS_DiagResp\nCAN DATA", "READ"=FALSE, "WRITE"=FALSE}, {"FUNCTION"="GS_WarnMsg\nCAN DATA", "READ"=FALSE, "WRITE"=FALSE}, {"FUNCTION"="GW_BCM_Immo_MHU_Byte\nCAN DATA", "READ"=FALSE, "WRITE"=FALSE}, {"FUNCTION"="GW_BCM_RemoteCtrlSts\nCAN DATA", "READ"=FALSE, "WRITE"=FALSE}, {"FUNCTION"="HOD_Heating\nCAN DATA", "READ"=FALSE, "WRITE"=FALSE}, {"FUNCTION"="HOD_Heating_FDBK\nCAN DATA", "READ"=FALSE, "WRITE"=FALSE}, {"FUNCTION"="HUD_DiagReq\nCAN DATA", "READ"=FALSE, "WRITE"=FALSE}, {"FUNCTION"="HUD_DiagResp\nCAN DATA", "READ"=FALSE, "WRITE"=FALSE}, {"FUNCTION"="HUD_ECU_Status\nCAN DATA", "READ"=FALSE, "WRITE"=FALSE}, {"FUNCTION"="HUD_NM\nCAN DATA", "READ"=FALSE, "WRITE"=FALSE}, {"FUNCTION"="HUD_State\nCAN DATA", "READ"=FALSE, "WRITE"=FALSE}, {"FUNCTION"="HUD_WarnMsg\nCAN DATA", "READ"=FALSE, "WRITE"=FALSE}, {"FUNCTION"="HUD_rDiagReq\nCAN DATA", "READ"=FALSE, "WRITE"=FALSE}, {"FUNCTION"="HUD_rDiagResp\nCAN DATA", "READ"=FALSE, "WRITE"=FALSE}, {"FUNCTION"="IC_BORD_COMP_TRIP_A\nCAN DATA", "READ"=FALSE, "WRITE"=FALSE}, {"FUNCTION"="IC_BORD_COMP_TRIP_Auto\nCAN DATA", "READ"=FALSE, "WRITE"=FALSE}, {"FUNCTION"="IC_BORD_COMP_TRIP_B\nCAN DATA", "READ"=FALSE, "WRITE"=FALSE}, {"FUNCTION"="IC_MILEAGE\nCAN DATA", "READ"=FALSE, "WRITE"=FALSE}, {"FUNCTION"="IC_ODO\nCAN DATA", "READ"=FALSE, "WRITE"=FALSE}, {"FUNCTION"="IC_RELATIVIME\nCAN DATA", "READ"=FALSE, "WRITE"=FALSE}, {"FUNCTION"="IC_SENSOR\nCAN DATA", "READ"=FALSE, "WRITE"=FALSE}, {"FUNCTION"="IC_STAT_AIRBAG\nCAN DATA", "READ"=FALSE, "WRITE"=FALSE}, {"FUNCTION"="IDB_ACC_LONG_LAT_YAW\nCAN DATA", "READ"=FALSE, "WRITE"=FALSE}, {"FUNCTION"="IDB_DiagReq\nCAN DATA", "READ"=FALSE, "WRITE"=FALSE}, {"FUNCTION"="IDB_DiagResp\nCAN DATA", "READ"=FALSE, "WRITE"=FALSE}, {"FUNCTION"="IDB_EPB_STATUS\nCAN DATA", "READ"=FALSE, "WRITE"=FALSE}, {"FUNCTION"="IDB_FUNCTION\nCAN DATA", "READ"=FALSE, "WRITE"=FALSE}, {"FUNCTION"="IDB_MILEAGE\nCAN DATA", "READ"=FALSE, "WRITE"=FALSE}, {"FUNCTION"="IDB_STATUS\nCAN DATA", "READ"=FALSE, "WRITE"=FALSE}, {"FUNCTION"="IDB_V_VEH\nCAN DATA", "READ"=FALSE, "WRITE"=FALSE}, {"FUNCTION"="IDB_WarnMsg\nCAN DATA", "READ"=FALSE, "WRITE"=FALSE}, {"FUNCTION"="LDML_LIGHT\nCAN DATA", "READ"=FALSE, "WRITE"=FALSE}, {"FUNCTION"="LDMR_LIGHT\nCAN DATA", "READ"=FALSE, "WRITE"=FALSE}, {"FUNCTION"="LDM_L_DiagReq\nCAN DATA", "READ"=FALSE, "WRITE"=FALSE}, {"FUNCTION"="LDM_L_DiagResp\nCAN DATA", "READ"=FALSE, "WRITE"=FALSE}, {"FUNCTION"="LDM_R_DiagReq\nCAN DATA", "READ"=FALSE, "WRITE"=FALSE}, {"FUNCTION"="LDM_R_DiagResp\nCAN DATA", "READ"=FALSE, "WRITE"=FALSE}, {"FUNCTION"="MFS_Control_Button\nCAN DATA", "READ"=FALSE, "WRITE"=FALSE}, {"FUNCTION"="MHU_ADAS_RP_Ctrl\nCAN DATA", "READ"=FALSE, "WRITE"=FALSE}, {"FUNCTION"="MHU_ADAS_RSSI\nCAN DATA", "READ"=FALSE, "WRITE"=FALSE}, {"FUNCTION"="MHU_ADAS_req\nCAN DATA", "READ"=FALSE, "WRITE"=FALSE}, {"FUNCTION"="MHU_AMP_Ann1_ModeSET\nCAN DATA", "READ"=FALSE, "WRITE"=FALSE}, {"FUNCTION"="MHU_AMP_Ann1_PromptsSET\nCAN DATA", "READ"=FALSE, "WRITE"=FALSE}, {"FUNCTION"="MHU_AMP_Ann2_SpeakerSET\nCAN DATA", "READ"=FALSE, "WRITE"=FALSE}, {"FUNCTION"="MHU_AmpEQType\nCAN DATA", "READ"=FALSE, "WRITE"=FALSE}, {"FUNCTION"="MHU_AmpSET\nCAN DATA", "READ"=FALSE, "WRITE"=FALSE}, {"FUNCTION"="MHU_Auth_Immo\nCAN DATA", "READ"=FALSE, "WRITE"=FALSE}, {"FUNCTION"="MHU_Auth_Immo_ADAS\nCAN DATA", "READ"=FALSE, "WRITE"=FALSE}, {"FUNCTION"="MHU_Avas_Setting\nCAN DATA", "READ"=FALSE, "WRITE"=FALSE}, {"FUNCTION"="MHU_BCM_Color_Req\nCAN DATA", "READ"=FALSE, "WRITE"=FALSE}, {"FUNCTION"="MHU_BCM_DoorsCtrl\nCAN DATA", "READ"=FALSE, "WRITE"=FALSE}, {"FUNCTION"="MHU_BCM_HornLightControl\nCAN DATA", "READ"=FALSE, "WRITE"=FALSE}, {"FUNCTION"="MHU_BCM_IntensityTiming_Req\nCAN DATA", "READ"=FALSE, "WRITE"=FALSE}, {"FUNCTION"="MHU_BCM_RemoteClampCtrl\nCAN DATA", "READ"=FALSE, "WRITE"=FALSE}, {"FUNCTION"="MHU_CCUF_ClimateSetting\nCAN DATA", "READ"=FALSE, "WRITE"=FALSE}, {"FUNCTION"="MHU_CCUR_ClimateSetting\nCAN DATA", "READ"=FALSE, "WRITE"=FALSE}, {"FUNCTION"="MHU_CPD_Confirm\nCAN DATA", "READ"=FALSE, "WRITE"=FALSE}, {"FUNCTION"="MHU_CarMode_Switch\nCAN DATA", "READ"=FALSE, "WRITE"=FALSE}, {"FUNCTION"="MHU_ComfortSetting\nCAN DATA", "READ"=FALSE, "WRITE"=FALSE}, {"FUNCTION"="MHU_DATE_TIME\nCAN DATA", "READ"=FALSE, "WRITE"=FALSE}, {"FUNCTION"="MHU_DIGIT_SPEED\nCAN DATA", "READ"=FALSE, "WRITE"=FALSE}, {"FUNCTION"="MHU_DMS_STATUS\nCAN DATA", "READ"=FALSE, "WRITE"=FALSE}, {"FUNCTION"="MHU_DRIVER_INFO\nCAN DATA", "READ"=FALSE, "WRITE"=FALSE}, {"FUNCTION"="MHU_DiagReq\nCAN DATA", "READ"=FALSE, "WRITE"=FALSE}, {"FUNCTION"="MHU_DiagResp\nCAN DATA", "READ"=FALSE, "WRITE"=FALSE}, {"FUNCTION"="MHU_DoorSetting\nCAN DATA", "READ"=FALSE, "WRITE"=FALSE}, {"FUNCTION"="MHU_EvSetting\nCAN DATA", "READ"=FALSE, "WRITE"=FALSE}, {"FUNCTION"="MHU_FEEDBACK_APA\nCAN DATA", "READ"=FALSE, "WRITE"=FALSE}, {"FUNCTION"="MHU_FOTA_ReqAll\nCAN DATA", "READ"=FALSE, "WRITE"=FALSE}, {"FUNCTION"="MHU_FOTA_STATUS\nCAN DATA", "READ"=FALSE, "WRITE"=FALSE}, {"FUNCTION"="MHU_HEADLAMP_CTL\nCAN DATA", "READ"=FALSE, "WRITE"=FALSE}, {"FUNCTION"="MHU_HUD_BASE\nCAN DATA", "READ"=FALSE, "WRITE"=FALSE}, {"FUNCTION"="MHU_HUD_Info_1\nCAN DATA", "READ"=FALSE, "WRITE"=FALSE}, {"FUNCTION"="MHU_HUD_NAV_DISP\nCAN DATA", "READ"=FALSE, "WRITE"=FALSE}, {"FUNCTION"="MHU_HUD_NAV_GuidanceCont\nCAN DATA", "READ"=FALSE, "WRITE"=FALSE}, {"FUNCTION"="MHU_HudPositionSetting\nCAN DATA", "READ"=FALSE, "WRITE"=FALSE}, {"FUNCTION"="MHU_HudSetting\nCAN DATA", "READ"=FALSE, "WRITE"=FALSE}, {"FUNCTION"="MHU_IDB_Mode_Select\nCAN DATA", "READ"=FALSE, "WRITE"=FALSE}, {"FUNCTION"="MHU_ISA_Speed\nCAN DATA", "READ"=FALSE, "WRITE"=FALSE}, {"FUNCTION"="MHU_LightSetting\nCAN DATA", "READ"=FALSE, "WRITE"=FALSE}, {"FUNCTION"="MHU_MirrorAdjust\nCAN DATA", "READ"=FALSE, "WRITE"=FALSE}, {"FUNCTION"="MHU_NAV_JUNC_INFO\nCAN DATA", "READ"=FALSE, "WRITE"=FALSE}, {"FUNCTION"="MHU_NM\nCAN DATA", "READ"=FALSE, "WRITE"=FALSE}, {"FUNCTION"="MHU_SEAT_CONTROL\nCAN DATA", "READ"=FALSE, "WRITE"=FALSE}, {"FUNCTION"="MHU_STATUS\nCAN DATA", "READ"=FALSE, "WRITE"=FALSE}, {"FUNCTION"="MHU_SeatVentHeat\nCAN DATA", "READ"=FALSE, "WRITE"=FALSE}, {"FUNCTION"="MHU_SteeringAdjust\nCAN DATA", "READ"=FALSE, "WRITE"=FALSE}, {"FUNCTION"="MHU_UserProfile\nCAN DATA", "READ"=FALSE, "WRITE"=FALSE}, {"FUNCTION"="MHU_WindowSetting\nCAN DATA", "READ"=FALSE, "WRITE"=FALSE}, {"FUNCTION"="MRGEN_DiagReq\nCAN DATA", "READ"=FALSE, "WRITE"=FALSE}, {"FUNCTION"="MRGEN_DiagResp\nCAN DATA", "READ"=FALSE, "WRITE"=FALSE}, {"FUNCTION"="OCS_P_DiagReq\nCAN DATA", "READ"=FALSE, "WRITE"=FALSE}, {"FUNCTION"="OCS_P_DiagResp\nCAN DATA", "READ"=FALSE, "WRITE"=FALSE}, {"FUNCTION"="POD_DCDC_DiagReq\nCAN DATA", "READ"=FALSE, "WRITE"=FALSE}, {"FUNCTION"="POD_DCDC_DiagResp\nCAN DATA", "READ"=FALSE, "WRITE"=FALSE}, {"FUNCTION"="POD_GW_Request\nCAN DATA", "READ"=FALSE, "WRITE"=FALSE}, {"FUNCTION"="POD_GW_Response\nCAN DATA", "READ"=FALSE, "WRITE"=FALSE}, {"FUNCTION"="POD_OBC_DiagReq\nCAN DATA", "READ"=FALSE, "WRITE"=FALSE}, {"FUNCTION"="POD_OBC_DiagResp\nCAN DATA", "READ"=FALSE, "WRITE"=FALSE}, {"FUNCTION"="POD_WarnMsg\nCAN DATA", "READ"=FALSE, "WRITE"=FALSE}, {"FUNCTION"="PSM_D_DiagReq\nCAN DATA", "READ"=FALSE, "WRITE"=FALSE}, {"FUNCTION"="PSM_D_DiagResp\nCAN DATA", "READ"=FALSE, "WRITE"=FALSE}, {"FUNCTION"="PSM_D_SEAT_CONTROL\nCAN DATA", "READ"=FALSE, "WRITE"=FALSE}, {"FUNCTION"="PSM_SEAT_POSITION\nCAN DATA", "READ"=FALSE, "WRITE"=FALSE}, {"FUNCTION"="PSM_WarnMsg\nCAN DATA", "READ"=FALSE, "WRITE"=FALSE}, {"FUNCTION"="RCU_DiagReq\nCAN DATA", "READ"=FALSE, "WRITE"=FALSE}, {"FUNCTION"="RCU_DiagResp\nCAN DATA", "READ"=FALSE, "WRITE"=FALSE}, {"FUNCTION"="RCU_WarnMsg\nCAN DATA", "READ"=FALSE, "WRITE"=FALSE}, {"FUNCTION"="SAS_Sensor\nCAN DATA", "READ"=FALSE, "WRITE"=FALSE}, {"FUNCTION"="SCAM_DiagReq\nCAN DATA", "READ"=FALSE, "WRITE"=FALSE}, {"FUNCTION"="SCAM_DiagResp\nCAN DATA", "READ"=FALSE, "WRITE"=FALSE}, {"FUNCTION"="SCM_Raw_Status\nCAN DATA", "READ"=FALSE, "WRITE"=FALSE}, {"FUNCTION"="SHVU_F_Confirm_Sts\nCAN DATA", "READ"=FALSE, "WRITE"=FALSE}, {"FUNCTION"="SHVU_F_DiagReq\nCAN DATA", "READ"=FALSE, "WRITE"=FALSE}, {"FUNCTION"="SHVU_F_DiagResp\nCAN DATA", "READ"=FALSE, "WRITE"=FALSE}, {"FUNCTION"="SHVU_R_Confirm_Sts\nCAN DATA", "READ"=FALSE, "WRITE"=FALSE}, {"FUNCTION"="SHVU_R_DiagReq\nCAN DATA", "READ"=FALSE, "WRITE"=FALSE}, {"FUNCTION"="SHVU_R_DiagResp\nCAN DATA", "READ"=FALSE, "WRITE"=FALSE}, {"FUNCTION"="SRR_FL_DiagReq\nCAN DATA", "READ"=FALSE, "WRITE"=FALSE}, {"FUNCTION"="SRR_FL_DiagResp\nCAN DATA", "READ"=FALSE, "WRITE"=FALSE}, {"FUNCTION"="SRR_FR_DiagReq\nCAN DATA", "READ"=FALSE, "WRITE"=FALSE}, {"FUNCTION"="SRR_FR_DiagResp\nCAN DATA", "READ"=FALSE, "WRITE"=FALSE}, {"FUNCTION"="SRR_RL_DiagReq\nCAN DATA", "READ"=FALSE, "WRITE"=FALSE}, {"FUNCTION"="SRR_RL_DiagResp\nCAN DATA", "READ"=FALSE, "WRITE"=FALSE}, {"FUNCTION"="SRR_RR_DiagReq\nCAN DATA", "READ"=FALSE, "WRITE"=FALSE}, {"FUNCTION"="SRR_RR_DiagResp\nCAN DATA", "READ"=FALSE, "WRITE"=FALSE}, {"FUNCTION"="SeatMassage_Input\nCAN DATA", "READ"=FALSE, "WRITE"=FALSE}, {"FUNCTION"="SeatMassage_Output\nCAN DATA", "READ"=FALSE, "WRITE"=FALSE}, {"FUNCTION"="Sensor_Fault\nCAN DATA", "READ"=FALSE, "WRITE"=FALSE}, {"FUNCTION"="TPMS_TirePressure\nCAN DATA", "READ"=FALSE, "WRITE"=FALSE}, {"FUNCTION"="TRM_DiagReq\nCAN DATA", "READ"=FALSE, "WRITE"=FALSE}, {"FUNCTION"="TRM_DiagResp\nCAN DATA", "READ"=FALSE, "WRITE"=FALSE}, {"FUNCTION"="TRM_WarnMsg\nCAN DATA", "READ"=FALSE, "WRITE"=FALSE}, {"FUNCTION"="VCU_ChargingConnection\nCAN DATA", "READ"=FALSE, "WRITE"=FALSE}, {"FUNCTION"="VCU_DiagReq\nCAN DATA", "READ"=FALSE, "WRITE"=FALSE}, {"FUNCTION"="VCU_DiagResp\nCAN DATA", "READ"=FALSE, "WRITE"=FALSE}, {"FUNCTION"="VCU_HMI_Info\nCAN DATA", "READ"=FALSE, "WRITE"=FALSE}, {"FUNCTION"="VCU_HV_DrvSys_status\nCAN DATA", "READ"=FALSE, "WRITE"=FALSE}, {"FUNCTION"="VCU_HVsystem_status\nCAN DATA", "READ"=FALSE, "WRITE"=FALSE}, {"FUNCTION"="VCU_MHU_info\nCAN DATA", "READ"=FALSE, "WRITE"=FALSE}, {"FUNCTION"="VCU_WarnMsg\nCAN DATA", "READ"=FALSE, "WRITE"=FALSE}, {"FUNCTION"="WLC_Status\nCAN DATA", "READ"=FALSE, "WRITE"=FALSE}, {"FUNCTION"="WLC_Status_2\nCAN DATA", "READ"=FALSE, "WRITE"=FALSE}, {"FUNCTION"="XGW_DiagReq\nCAN DATA", "READ"=FALSE, "WRITE"=FALSE}, {"FUNCTION"="XGW_DiagResp\nCAN DATA", "READ"=FALSE, "WRITE"=FALSE}, {"FUNCTION"="XGW_FOTA_StsConfirm\nCAN DATA", "READ"=FALSE, "WRITE"=FALSE}, {"FUNCTION"="XGW_HCMInfo\nCAN DATA", "READ"=FALSE, "WRITE"=FALSE}, {"FUNCTION"="XGW_Info_Collect\nCAN DATA", "READ"=FALSE, "WRITE"=FALSE}, {"FUNCTION"="XGW_NM\nCAN DATA", "READ"=FALSE, "WRITE"=FALSE}, {"FUNCTION"="XGW_System_Info\nCAN DATA", "READ"=FALSE, "WRITE"=FALSE}, {"FUNCTION"="XGW_WarnMsg\nCAN DATA", "READ"=FALSE, "WRITE"=FALSE}, {"FUNCTION"="YSS_DiagReq\nCAN DATA", "READ"=FALSE, "WRITE"=FALSE}, {"FUNCTION"="YSS_DiagResp\nCAN DATA", "READ"=FALSE, "WRITE"=FALSE}]  # ALL DBC FUNCTIONS
        w153 = T8 {"Current VI Reference"=refnum, "Close Panel on Exit?"=FALSE}  # Core
        w155 = TRUE  # Your Boolean data
        w154 = ""  # Your string data
        # "do not delete - used by framework"
        # "Data names and types of shift register data are defined by this bundle."
        # "Initialize the shift-register data, here.\n(data names are defined by what you wire into the bundle function)"
        n66 = Bundle("Core"=w153, "Your Boolean data"=w155, "Your string data"=w154, "ALL DBC FUNCTIONS"=w152, "File paths"=w151, "DBC FUNCTIONS"=w150) -> (w157:T6)  [unwired: 1 in]
        n67 = call <vilib>:"Add State(s) to Queue__JKI_lib_State_Machine.vi"("State(s) in (\"\")"=w159) -> ("States Out"=w158:string)  [unwired: 14 in]
      }
      frame "Data: Cleanup" {
        # "Cleanup any data and references, here.\n(this is called automatically, by the Macro: Exit)"
        n68 = Unbundle By Name(w160) -> ("Core.Current VI Reference"=w163:refnum<vi>)
        n69 = Close Reference(reference=w163, error in (no error)=w162) -> (error out=w161:errorcluster)
        n70 = call <vilib>:"Add State(s) to Queue__JKI_lib_State_Machine.vi"("State(s) in (\"\")"=w165) -> ("States Out"=w164:string)  [unwired: 14 in]
      }
      frame "---------- Events ----------" {
        # "Do not put any code in this frame.\n(It is a separator no-op. You can make a copy of this frame to create a new UI frame)"
        n71 = call <vilib>:"Add State(s) to Queue__JKI_lib_State_Machine.vi"("State(s) in (\"\")"=w169) -> ("States Out"=w168:string)  [unwired: 14 in]
      }
      frame "Events: Register" {
        # "Do not put any code in this frame.\n(It is a separator no-op. You can make a copy of this frame to create a new UI frame)"
        n72 = call <vilib>:"Add State(s) to Queue__JKI_lib_State_Machine.vi"("State(s) in (\"\")"=w173) -> ("States Out"=w172:string)  [unwired: 14 in]
      }
      frame "Events: Unregister" {
        # "Do not put any code in this frame.\n(It is a separator no-op. You can make a copy of this frame to create a new UI frame)"
        n73 = Unregister For Events(event registration refnum=w176, error in=w175) -> (error out=w174:errorcluster)
        n74 = call <vilib>:"Add State(s) to Queue__JKI_lib_State_Machine.vi"("State(s) in (\"\")"=w179) -> ("States Out"=w178:string)  [unwired: 14 in]
      }
      frame "---------- UI ----------" {
        # "Do not put any code in this frame.\n(It is a separator no-op. You can make a copy of this frame to create a new UI frame)"
        n75 = call <vilib>:"Add State(s) to Queue__JKI_lib_State_Machine.vi"("State(s) in (\"\")"=w183) -> ("States Out"=w182:string)  [unwired: 14 in]
      }
      frame "UI: Initialize" {
        # "Initialize the User Interface, here.\n(this is called automatically, by the Macro: Init)"
        n76 = invoke class="VI" method="Default Vals.Reinit All"(error in=w186) -> (error out=w185:errorcluster)  [unwired: 2 in, 2 out]
        n77 = Current VI's Path() -> (path=w192:path)
        n78 = call "FEV_Strip & Build Path.vi"("Strip Levels"=2, "error in (no error)"=w185, "Build Path"="Data\\Models", "Path In"=w192) -> ("error out"=w190:errorcluster, "New Path Out"=w187:path)  [unwired: 5 in, 1 out]
        n79 = Bundle By Name(cluster=w189, "File paths.Base file path"=w187) -> (w188:T6)
        n80 = call <vilib>:"Add State(s) to Queue__JKI_lib_State_Machine.vi"("State(s) in (\"\")"=w195) -> ("States Out"=w194:string)  [unwired: 14 in]
        "Headline" <- "CAN Configuration" ("Headline")
      }
      frame "UI: Cursor Set" {
        # "Argument"
        # "Set and Unset Cursor Busy.\n(Usage: \"UI: Cursor Set >> Busy|Idle\")"
        n81 = case shown="\"Idle\", Default" w196 {
          tunnel: w198 -> [w203 w205]
          tunnel: [w202 w204] -> w197
          frame "Idle", Default {
            n82 = call <vilib>:"Unset Busy.vi"("error in (no error)"=w203) -> ("error out"=w202:errorcluster)  [unwired: 10 in]
          }
          frame "Busy" {
            n83 = call <vilib>:"Set Busy.vi"("error in (no error)"=w205) -> ("error out"=w204:errorcluster)  [unwired: 9 in, 1 out]
          }
        }
        n84 = call <vilib>:"Add State(s) to Queue__JKI_lib_State_Machine.vi"("State(s) in (\"\")"=w201) -> ("States Out"=w200:string)  [unwired: 14 in]
      }
      frame "UI: Front Panel State" {
        # "Argument"
        # "Set Front Panel Open or Closed\n(Usage: \"UI: Front Panel State >> Open|Close\")"
        n85 = Unbundle By Name(w208) -> ("Core.Current VI Reference"=w207:refnum<vi>)
        n86 = case shown="\"Open\", \"Standard\", Default" w206 {
          tunnel: w210 -> [w218 w233 w244 w257 w270]
          tunnel: [w220 w234 w246 w259 w272] -> w209
          tunnel: w207 -> [w219 w231 w245 w258 w271]
          frame "Open", "Standard", Default {
            w213 = T4."Standard" ("State")
            n87 = property class="VI"(reference=w219, error in=w218) -> (reference out=w216:refnum<vi>, error out=w217:errorcluster, "FP.State"=w215:T4)
            n88 = Not Equal?(x=w215, y=w213) -> (x != y?=w214:bool)
            n89 = case shown="True" w214 {
              tunnel: [w224 w226] -> w220
              tunnel: w217 -> [w223 w226]
              tunnel: w216 -> [w222 _]
              tunnel: w213 -> [w221 _]
              frame True {
                n90 = invoke class="VI" method="FP.Open"(reference=w222, error in=w223, "Activate"=TRUE, "State"=w221) -> (error out=w224:errorcluster)  [unwired: 1 in, 4 out]
              }
              frame False {
              }
            }
          }
          frame "Close", "Closed" {
            n91 = property class="VI"(reference=w231, error in=w233) -> (reference out=w230:refnum<vi>, error out=w232:errorcluster, "FP.State"=w228:T4)
            n92 = Not Equal?(x=w228, y=T4."Closed" ("Front Panel Window:State")) -> (x != y?=w227:bool)
            n93 = case shown="True" w227 {
              tunnel: [w235 w238] -> w234
              tunnel: w232 -> [w235 w237]
              tunnel: w230 -> [_ w236]
              frame False {
              }
              frame True {
                n94 = invoke class="VI" method="FP.Close"(reference=w236, error in=w237) -> (error out=w238:errorcluster)  [unwired: 1 in, 2 out]
              }
            }
          }
          frame "Hidden", "Hide" {
            w239 = T4."Hidden" ("State")
            n95 = property class="VI"(reference=w245, error in=w244) -> (reference out=w242:refnum<vi>, error out=w243:errorcluster, "FP.State"=w241:T4)
            n96 = Not Equal?(x=w241, y=w239) -> (x != y?=w240:bool)
            n97 = case shown="True" w240 {
              tunnel: [w250 w251] -> w246
              tunnel: w243 -> [w249 w251]
              tunnel: w242 -> [w248 _]
              tunnel: w239 -> [w247 _]
              frame True {
                n98 = invoke class="VI" method="FP.Open"(reference=w248, error in=w249, "State"=w247) -> (error out=w250:errorcluster)  [unwired: 2 in, 4 out]
              }
              frame False {
              }
            }
          }
          frame "Minimize", "Minimized" {
            w252 = T4."Minimized" ("State")
            n99 = property class="VI"(reference=w258, error in=w257) -> (reference out=w255:refnum<vi>, error out=w256:errorcluster, "FP.State"=w254:T4)
            n100 = Not Equal?(x=w254, y=w252) -> (x != y?=w253:bool)
            n101 = case shown="True" w253 {
              tunnel: [w263 w264] -> w259
              tunnel: w256 -> [w262 w264]
              tunnel: w255 -> [w261 _]
              tunnel: w252 -> [w260 _]
              frame True {
                n102 = invoke class="VI" method="FP.Open"(reference=w261, error in=w262, "State"=w260) -> (error out=w263:errorcluster)  [unwired: 2 in, 4 out]
              }
              frame False {
              }
            }
          }
          frame "Maximize", "Maximized" {
            w265 = T4."Maximized" ("State")
            n103 = property class="VI"(reference=w271, error in=w270) -> (reference out=w268:refnum<vi>, error out=w269:errorcluster, "FP.State"=w267:T4)
            n104 = Not Equal?(x=w267, y=w265) -> (x != y?=w266:bool)
            n105 = case shown="True" w266 {
              tunnel: [w276 w277] -> w272
              tunnel: w269 -> [w275 w277]
              tunnel: w268 -> [w274 _]
              tunnel: w265 -> [w273 _]
              frame True {
                n106 = invoke class="VI" method="FP.Open"(reference=w274, error in=w275, "State"=w273) -> (error out=w276:errorcluster)  [unwired: 2 in, 4 out]
              }
              frame False {
              }
            }
          }
        }
        n107 = call <vilib>:"Add State(s) to Queue__JKI_lib_State_Machine.vi"("State(s) in (\"\")"=w212) -> ("States Out"=w211:string)  [unwired: 14 in]
      }
      frame "---------- Macro ----------" {
        # "Do not put any code in this frame.\n(It is a separator no-op. You can make a copy of this frame to create a new Macro frame)"
        n108 = call <vilib>:"Add State(s) to Queue__JKI_lib_State_Machine.vi"("State(s) in (\"\")"=w281) -> ("States Out"=w280:string)  [unwired: 14 in]
      }
      frame "Macro: Initialize" {
        # "Initialization Macro\n(This is called once, when the VI starts)"
        n109 = call <vilib>:"Add State(s) to Queue__JKI_lib_State_Machine.vi"("State(s) in Front (\"\")"="Data: Initialize\nInitialize Core Data\nEvents: Register\nUI: Initialize\nUI: Front Panel State >> Open", "State(s) in (\"\")"=w286) -> ("States Out"=w285:string)  [unwired: 13 in]
      }
      frame "Macro: Exit" {
        # "Exit Macro\n(This is called once, when the VI exits)"
        n110 = Unbundle By Name(w293) -> ("Core.Close Panel on Exit?"=w292:bool)
        n111 = Select(t="UI: Front Panel State >> Close", s=w292, f="") -> (s? t:f=w289:string)
        n112 = call <vilib>:"Add State(s) to Queue__JKI_lib_State_Machine.vi"("State(s) in (\"\")"=w289, "State(s) at Back (\"\")"="Data: Cleanup\nEvents: Unregister\nExit") -> ("States Out"=w287:string)  [unwired: 13 in]
        n113 = call <vilib>:"Add State(s) to Queue__JKI_lib_State_Machine.vi"("State(s) in Front (\"\")"=w287, "State(s) in (\"\")"=w296) -> ("States Out"=w295:string)  [unwired: 13 in]
      }
      frame "---------- DATABSE ----------" {
        # "Template Separator\n(You can make a copy of, or modify, this frame)"
        n114 = call <vilib>:"Add State(s) to Queue__JKI_lib_State_Machine.vi"("State(s) in (\"\")"=w300) -> ("States Out"=w299:string)  [unwired: 14 in]
      }
      frame "DATABASE: SAVE DATABASE" {
        # "Your code here.\n(You can make a copy of, or modify, this frame)"
        n115 = Unbundle By Name(w312) -> ("DBC FUNCTIONS"=w303:T1[], "ALL DBC FUNCTIONS"=w308:T3[], "File paths.Model File path"=w306:path)
        n116 = Build Path(base path=w306, name or relative path="ALL DBC.txt") -> (appended path=w309:path)
        n117 = Build Path(base path=w306, name or relative path="DBC FUNCTION.txt") -> (appended path=w304:path)
        n118 = Write to Binary File(file (use dialog)=w309, data=w308, error in=w311) -> (error out=w307:errorcluster)  [unwired: 3 in, 2 out]
        n119 = Write to Binary File(file (use dialog)=w304, data=w303, error in=w307) -> (error out=w301:errorcluster)  [unwired: 3 in, 2 out]
        n120 = flat-sequence {
          tunnel: [w316] -> w302
          tunnel: w301 -> [w316]
          frame #0 {
            n121 = One Button Dialog(message="DBC data is Saved") -> ()  [unwired: 1 in, 1 out]
          }
        }
        n122 = call <vilib>:"Add State(s) to Queue__JKI_lib_State_Machine.vi"("State(s) in (\"\")"=w314) -> ("States Out"=w313:string)  [unwired: 14 in]
      }
      frame "DATABASE: READ DATABASE" {
        # "Your code here.\n(You can make a copy of, or modify, this frame)"
        n123 = Unbundle By Name(w333) -> ("DBC FUNCTIONS"=w318:T1[], "ALL DBC FUNCTIONS"=w334:T3[], "File paths.Model File path"=w324:path)
        n124 = Build Path(base path=w324, name or relative path="DBC FUNCTION.txt") -> (appended path=w323:path)
        n125 = Build Path(base path=w324, name or relative path="ALL DBC.txt") -> (appended path=w329:path)
        n126 = call <vilib>:"Check if File or Folder Exists.vi"("error in (no error)"=w322, "path"=w323) -> ("error out"=w321:errorcluster, "file or folder exists?"=w319:bool, "dup path"=w320:path)  [unwired: 7 in]
        n127 = call <vilib>:"Check if File or Folder Exists.vi"("error in (no error)"=w322, "path"=w329) -> ("error out"=w327:errorcluster, "file or folder exists?"=w326:bool, "dup path"=w328:path)  [unwired: 7 in]
        n128 = case shown="True" w326 {
          tunnel: w334 -> [w347 w353]
          tunnel: [w346 w351] -> w331
          tunnel: [w347 w350] -> w330
          tunnel: w328 -> [_ w349]
          tunnel: w327 -> [w346 w348]
          frame False {
          }
          frame True {
            n129 = Read from Binary File(5:w353, 8:w348, 11:w349) -> (0:w352:errorcluster, 2:w350:T3[])  [unwired: 3 in, 2 out]
            n130 = property on="ALL DBC FUNCTIONS" class="Arr (strict)"(error in=w352, "Value"=w350) -> (error out=w351:errorcluster)  [unwired: 1 in, 1 out]
          }
        }
        n131 = case shown="True" w319 {
          tunnel: w318 -> [w339 w345]
          tunnel: [w338 w341] -> _
          tunnel: [w339 w340] -> w317
          tunnel: w320 -> [_ w344]
          tunnel: w321 -> [w338 w343]
          frame False {
          }
          frame True {
            n132 = Read from Binary File(5:w345, 8:w343, 11:w344) -> (0:w342:errorcluster, 2:w340:T1[])  [unwired: 3 in, 2 out]
            n133 = property on="DBC FUNCTIONS" class="Arr (strict)"(error in=w342, "Value"=w340) -> (error out=w341:errorcluster)  [unwired: 1 in, 1 out]
          }
        }
        n134 = Bundle By Name(cluster=w333, "ALL DBC FUNCTIONS"=w330, "DBC FUNCTIONS"=w317) -> (w332:T6)
        n135 = call <vilib>:"Add State(s) to Queue__JKI_lib_State_Machine.vi"("State(s) in (\"\")"=w337) -> ("States Out"=w336:string)  [unwired: 14 in]
      }
    }
  }
